vi "Jenkins - Get Build status.vi"(8 "error in (no error)":errorcluster, 10 "Script Job Name (Within Build Script Folder)":string, 11 "IP Address":string) -> (0 "error out":errorcluster, 3 "Done?":bool, 5 "Text":string)   [LabVIEW 2014]
uses:
  <vilib>/Utility/error.llb/Error Cluster From Error Code.vi
  <vilib>/ErrorRing/Error Ring.xnode
  <vilib>/httpClient/LabVIEWHTTPClient.lvlib
  <vilib>/wsapi/NI_WebServices.lvlib
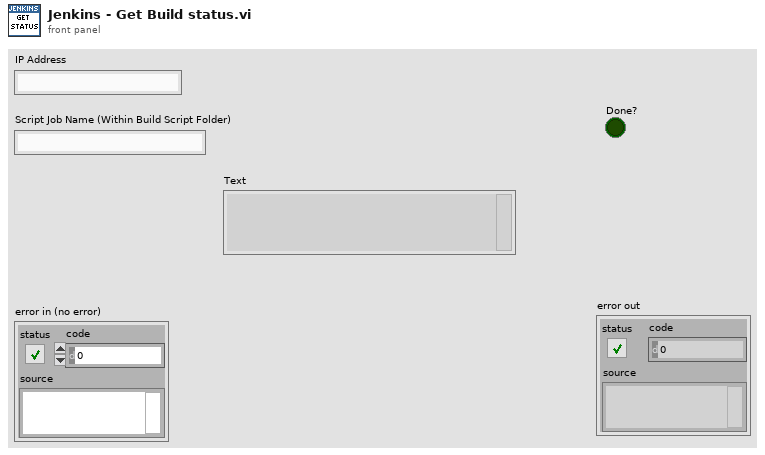
[diagram p1: front panel]
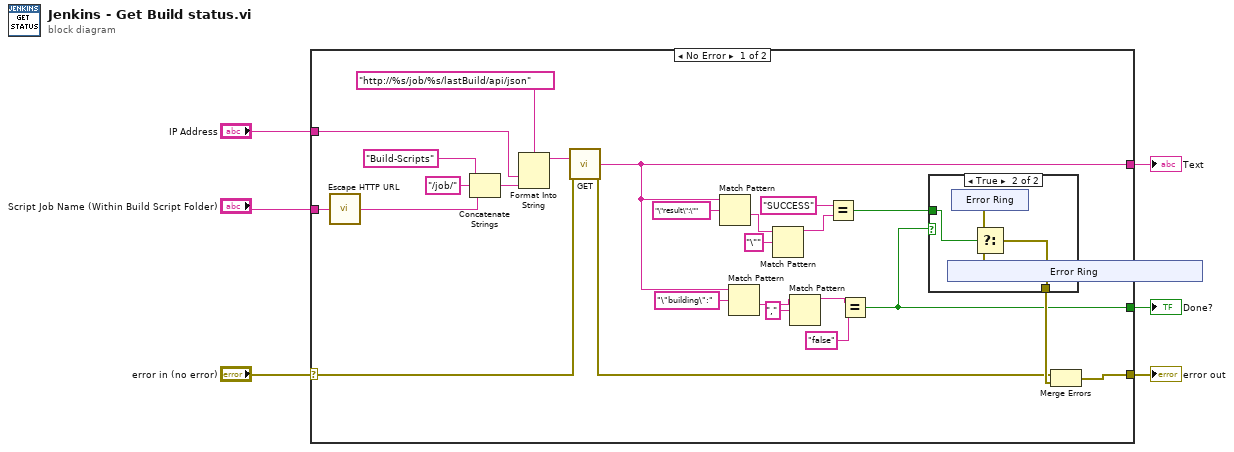
[diagram p0: block diagram]
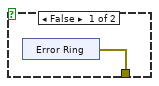
[diagram p2: hidden frame]
diagram:
  n1 = case shown="No Error" "error in (no error)" {
    selector: "error in (no error)" -> [w24 w44]
    tunnel: "IP Address" -> [w27 _]
    tunnel: "Script Job Name (Within Build Script Folder)" -> [w26 _]
    tunnel: [w8 w44] -> w4
    tunnel: [w18 _] -> w2
    tunnel: [w7 _] -> w1
    frame No Error {
      n2 = call <vilib>:"Escape HTTP URL.vi"("unescaped string in"=w26) -> ("escaped string out"=w25:string)
      n3 = Concatenate Strings("Build-Scripts" ("JSON"), "/job/" ("string"), w25) -> (w28:string)
      n4 = Format Into String(format string="http://%s/job/%s/lastBuild/api/json", w27, w28) -> (resulting string=w31:string)  [unwired: 2 in, 1 out]
      n5 = call <vilib>:"GET.vi"("url"=w31, "error in (no error)"=w24) -> ("body"=w18:string, "error out"=w9:errorcluster)  [unwired: 10 in, 2 out]
      n6 = Match Pattern(string=w18, regular expression="\"result\":\"") -> (after substring=w21:string)  [unwired: 1 in, 3 out]
      n7 = Match Pattern(string=w18, regular expression="\"building\":") -> (after substring=w15:string)  [unwired: 1 in, 3 out]
      n8 = Match Pattern(string=w21, regular expression="\"") -> (before substring=w13:string)  [unwired: 1 in, 3 out]
      n9 = Match Pattern(string=w15, regular expression=",") -> (before substring=w14:string)  [unwired: 1 in, 3 out]
      n10 = Equal?(x="SUCCESS", y=w13) -> (x = y?=w11:bool)
      n11 = Equal?(x=w14, y="false") -> (x = y?=w7:bool)
      n12 = case shown="True" w7 {
        tunnel: w11 -> [_ w37]
        tunnel: [w32 w34] -> w10
        frame False {
          n13 = xnode "Error Ring"() -> ("error out"=w32:errorcluster)
        }
        frame True {
          n14 = xnode "Error Ring"() -> ("error out"=w35:errorcluster)
          n15 = xnode "Error Ring"() -> ("error out"=w36:errorcluster)
          n16 = Select(t=w36, s=w37, f=w35) -> (s? t:f=w34:errorcluster)
        }
      }
      n17 = Merge Errors(w9, w10) -> (w8:errorcluster)
    }
    frame Error {
    }
  }
  "error out" <- w4
  "Text" <- w2
  "Done?" <- w1
